vi "7_Hole_Probe Pressures to UVW.vi"() -> ()   [LabVIEW 2017]
uses:
  Controls/Setup.ctl
  Globals/Meas_global.vi
panel:
  out "UVW":dbl[][](array[numeric])
  out "7 Hole Probe chs":string[](array[string])
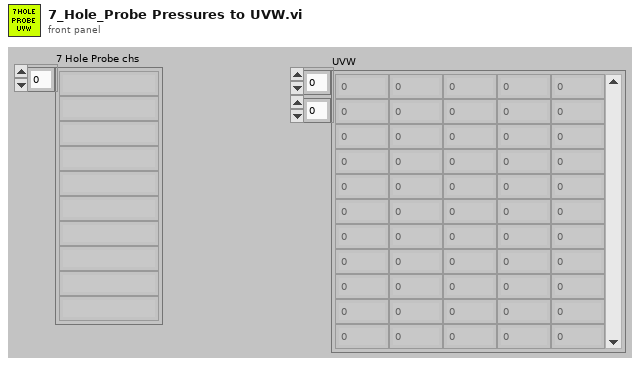
[diagram p1: front panel]
types:
  T1 = typedef "Analysis_info_cluster.ctl" = cluster{"Colour":u32, "Inst type":T2, "Inst name":string, "Symbol":string, "Code name":string, "Extra Info":string, "Inst Array":T3, "Extra Titles":string[], "Extra Values":string[], "U":dbl, "u^2":dbl, "u^3":dbl, "u^4":dbl, "Skew_u":dbl, "Kurt_u":dbl, "Sd Error in Mean":dbl, "% u'/U":dbl, "X":dbl, "Y":dbl, "Z":dbl, "Timescale integral Estimate":dbl, "Sd Error in Variance":dbl, "Calib File":path, "Calib Constants":dbl[], "Output Position":bool, "Full Stats":bool, "Av Sampling Rate":dbl, "Av No of Samples":dbl, "Total Meas Time (s)":dbl, "ADAM Ch Name":string, "Max value":dbl, "Min value":dbl, "Req Sample Rate Hz":dbl, "Sync Delay Time (s)":dbl, "Ch No":i16, "Device ID":string, "Use Latest Calib":bool, "Port":string}
  T2 = typedef "Inst_type.ctl" = enum16{"Propeller anemometer", "Raw voltage", "Pressure Transducer", "Pitot-static tube", "Preston tube", "Hot wire", "Cross wire 1", "Cross wire 2", "Generic Linear", "Generic Polynomial", "Generic BackPoly", "Fast FID", "Thermocouple", "Cold wire", "Pulsed Wire", "LDA Vel", "LDA Tran time", "LDA Arr time", "Microphone"}
  T3 = typedef "Instrument_Array.ctl" = enum16{"PWA", "LDA", "Analogue"}
  T4 = typedef "Time_Trace_Cluster.ctl" = cluster{"Weighting":dbl[], "Time (s)":dbl[], "Voltage":dbl[], "Eng Values":dbl[]}
  T5 = typedef "Setup.ctl" = enum16{"Run Program", "Show Setup", "Save Current Setup", "Setup Front Panel"}
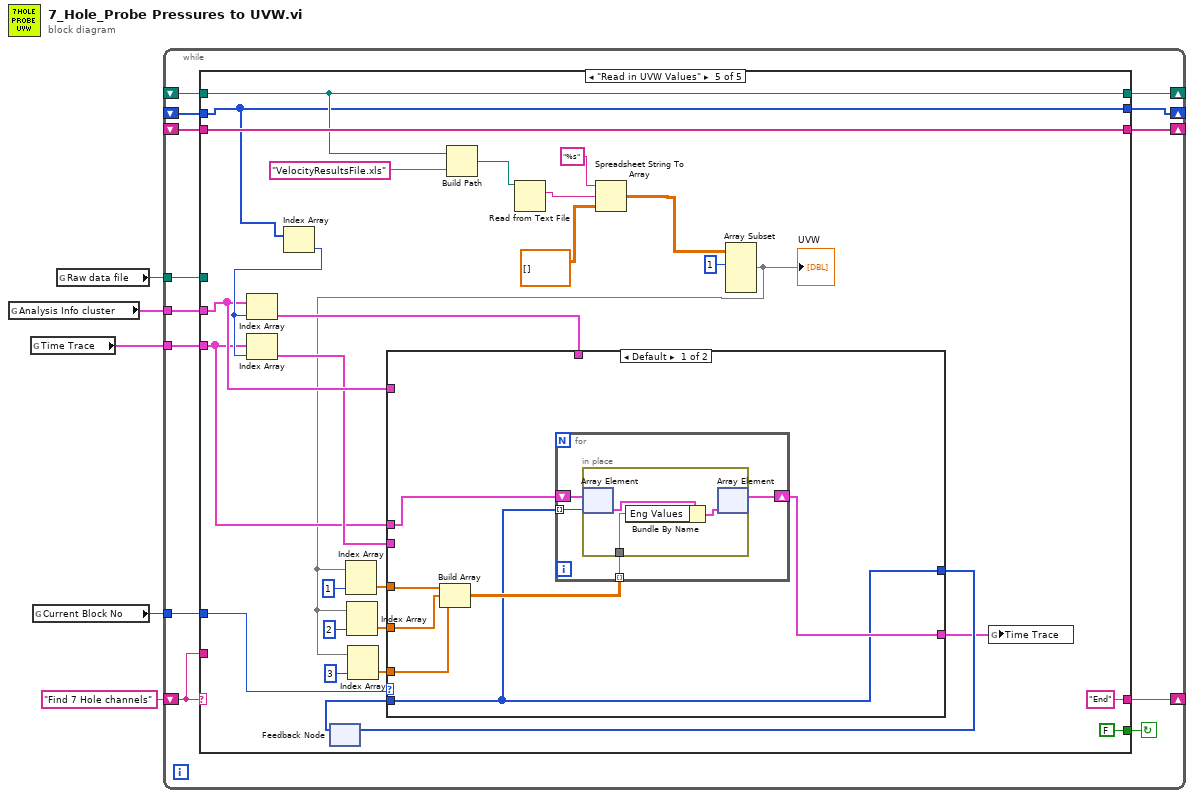
[diagram p0: block diagram]
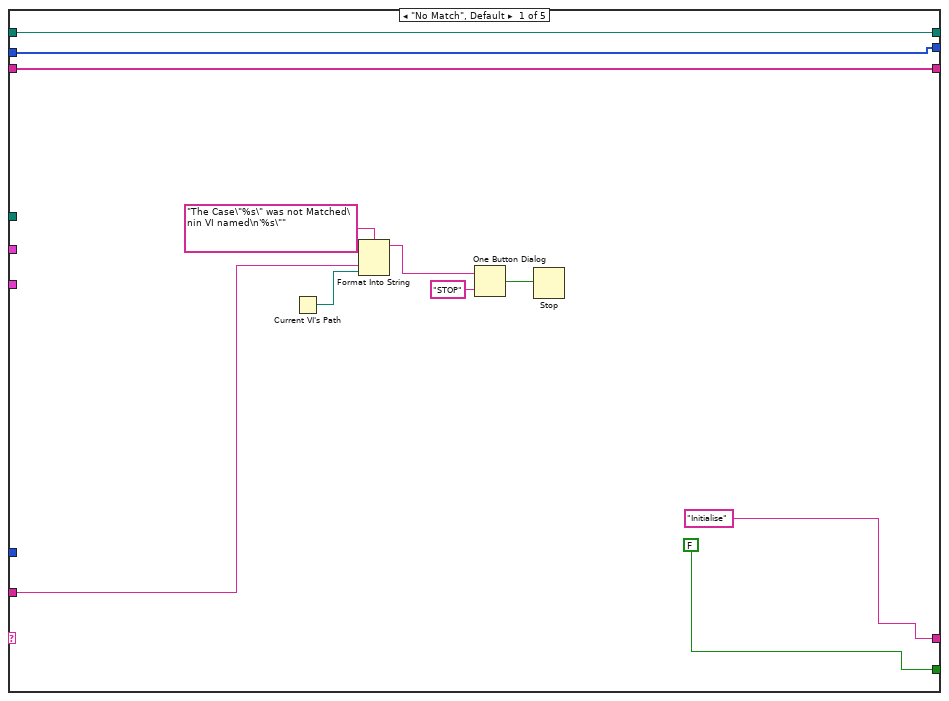
[diagram p2: hidden frame]
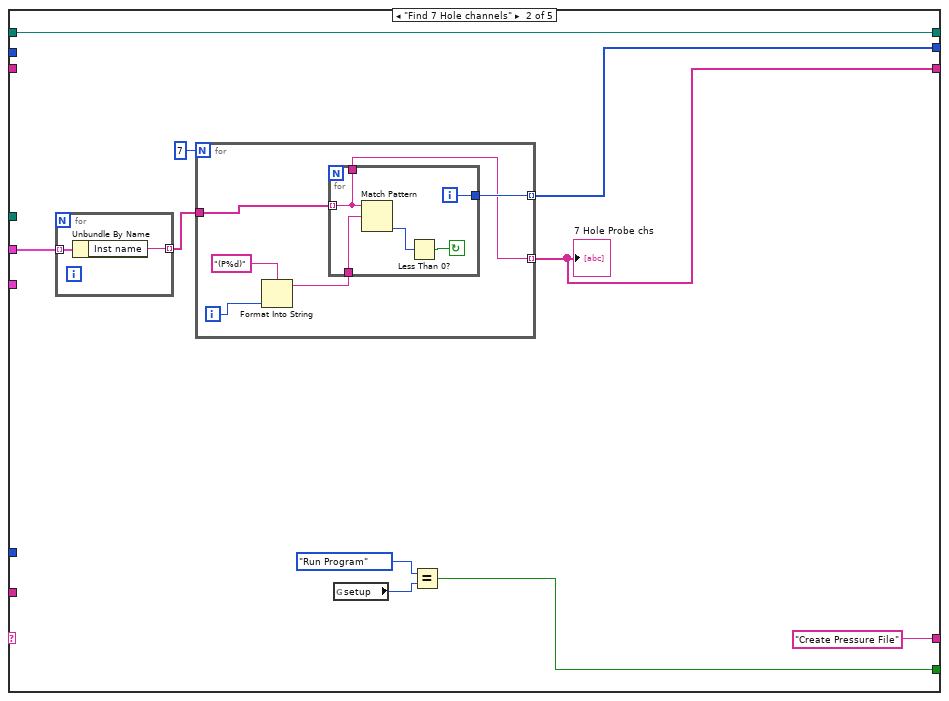
[diagram p3: hidden frame]
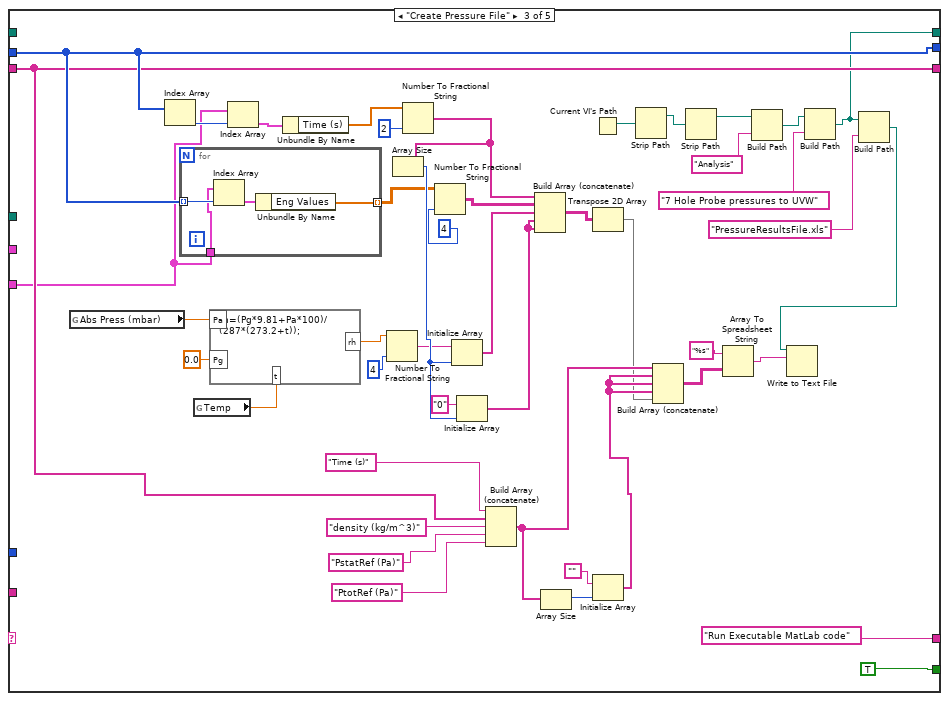
[diagram p4: hidden frame]
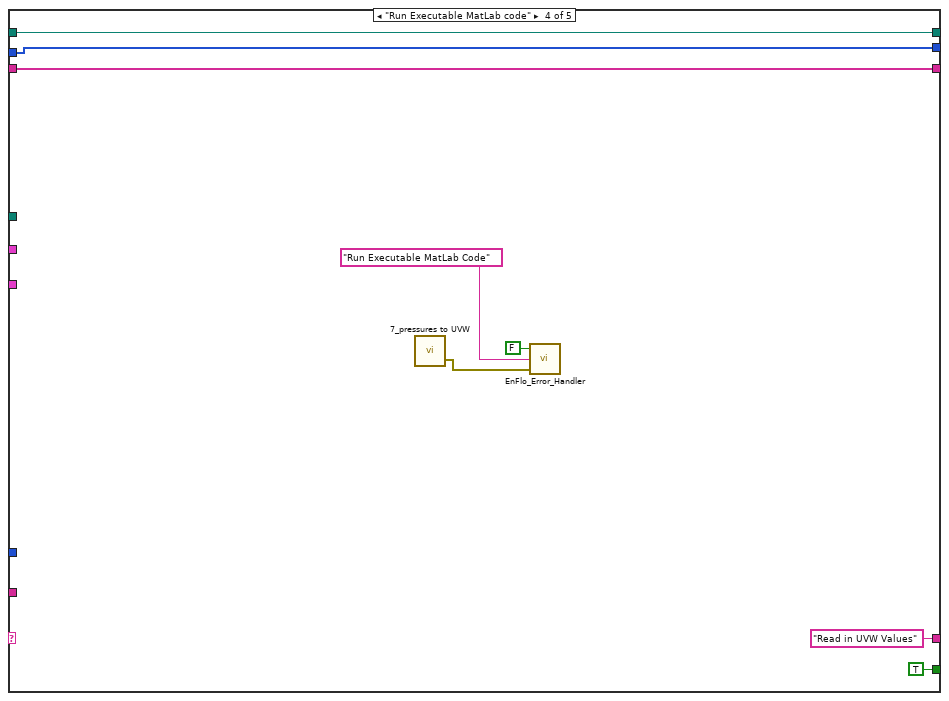
[diagram p5: hidden frame]
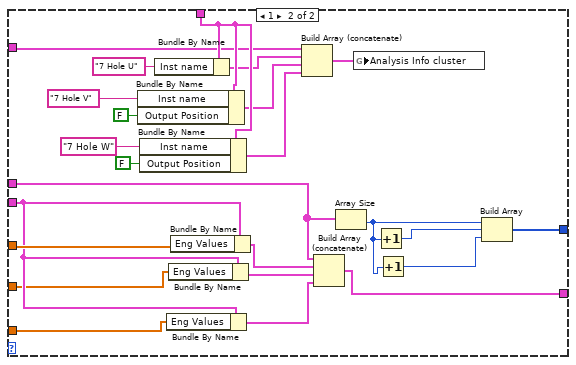
[diagram p6: hidden frame]
diagram:
  n1 = global read "Meas_global.vi" "Analysis Info cluster"() -> (w3:T1[])
  n2 = global read "Meas_global.vi" "Time Trace"() -> (w2:T4[])
  n3 = global read "Meas_global.vi" "Current Block No"() -> (w1:i32)
  n4 = global read "Meas_global.vi" "Raw data file"() -> (w4:path)
  n5 = while {
    shift-left: "Find 7 Hole channels" -> [w16]
    shift-right: [w17] -> _
    tunnel: w4 -> [w15]
    tunnel: w3 -> [w14]
    shift-right: [w13] -> _
    shift-left: _ -> [w12]
    shift-right: [w11] -> _
    shift-left: _ -> [w10]
    shift-right: [w9] -> _
    shift-left: _ -> [w8]
    tunnel: w2 -> [w7]
    tunnel: w1 -> [w6]
    stop <- w18 continue-if-true
    n6 = case shown="\"Read in UVW Values\"" w16 {
      tunnel: [FALSE w30 TRUE TRUE FALSE] -> w18
      tunnel: ["Initialise" "Create Pressure File" ("t") "Run Executable MatLab code" ("t") "Read in UVW Values" ("t") "End" ("t")] -> w17
      tunnel: w16 -> [w24 _ _ _ _]
      tunnel: w15 -> [_ _ _ _ _]
      tunnel: w14 -> [_ w39 _ _ w125]
      tunnel: [w21 w36 w95 w109 w132] -> w13
      tunnel: w12 -> [w21 _ w95 w109 w132]
      tunnel: [w20 w34 w68 w108 w137] -> w11
      tunnel: w10 -> [w20 _ w68 w108 w137]
      tunnel: [w19 w33 w54 w105 w134] -> w9
      tunnel: w8 -> [w19 w33 _ w105 w134]
      tunnel: w7 -> [_ _ w53 _ w115]
      tunnel: w6 -> [_ _ _ _ w114]
      frame "No Match", Default {
        n7 = Current VI's Path() -> (path=w23:path)
        n8 = Format Into String(format string="The Case\"%s\" was not Matched\nin VI named\n'%s\"" ("Format String"), w24, w23) -> (resulting string=w27:string)  [unwired: 2 in, 1 out]
        n9 = One Button Dialog(message=w27, button name ("OK")="STOP") -> (true=w25:bool)
        n10 = Stop(stop? (T)=w25) -> ()
      }
      frame "Find 7 Hole channels" {
        n11 = for {
          tunnel: w39 -> [w52] mode=indexing
          tunnel: [w51] -> w37 mode=indexing
          n12 = Unbundle By Name(w52) -> ("Inst name"=w51:string)
        }
        n13 = for {
          N: 7 -> [_]
          tunnel: w37 -> [w43]
          tunnel: [w41] -> w36 mode=indexing
          tunnel: [w40] -> w34 mode=indexing
          i -> [w45]
          n14 = Format Into String(format string="(P%d)", w45) -> (resulting string=w42:string)  [unwired: 2 in, 1 out]
          n15 = for {
            tunnel: w43 -> [w46] mode=indexing
            tunnel: w42 -> [w50]
            tunnel: [w47] -> w41
            tunnel: [w46] -> w40
            i -> [w47]
            stop <- w49 continue-if-true
            n16 = Match Pattern(string=w46, regular expression=w50) -> (offset past match=w48:i32)  [unwired: 1 in, 3 out]
            n17 = Less Than 0?(x=w48) -> (x < 0?=w49:bool)
          }
        }
        "7 Hole Probe chs" <- w34
        n18 = global read "Meas_global.vi" "setup"() -> (w32:T5)
        n19 = Equal?(x=Setup."Run Program" ("setup"), y=w32) -> (x = y?=w30:bool)
      }
      frame "Create Pressure File" {
        n20 = global read "Meas_global.vi" "Abs Press (mbar)"() -> (w91:dbl)
        n21 = Index Array(array=w95) -> (element=w93:i32)  [unwired: 1 in]
        n22 = for {
          tunnel: w95 -> [w101] mode=indexing
          tunnel: [w98] -> w77 mode=indexing
          tunnel: w53 -> [w99]
          n23 = Index Array(array=w99, index=w101) -> (element=w100:T4)
          n24 = Unbundle By Name(w100) -> ("Eng Values"=w98:dbl[])
        }
        n25 = global read "Meas_global.vi" "Temp"() -> (w92:dbl)
        n26 = formula code="rh=(Pg*9.81+Pa*100)/\n(287*(273.2+t));"("t"=w92, "Pg"=0.0 ("input variable"), "Pa"=w91) -> ("rh"=w74:dbl)
        n27 = Index Array(array=w53, index=w93) -> (element=w94:T4)
        n28 = Unbundle By Name(w94) -> ("Time (s)"=w81:dbl[])
        n29 = Number To Fractional String(number=w74, precision (6)=i16 4) -> (F-format string=w73:string)  [unwired: 2 in]
        n30 = Number To Fractional String(number=w81, precision (6)=i16 2) -> (F-format string=w79:string[])  [unwired: 2 in]
        n31 = Array Size(array=w79) -> (size(s)=w89:i32)
        n32 = Number To Fractional String(number=w77, precision (6)=i16 4) -> (F-format string=w76:string[][])  [unwired: 2 in]
        n33 = Initialize Array(w73, w89) -> (w87:string[])
        n34 = Initialize Array("0" ("element"), w89) -> (w86:string[])
        n35 = Build Array (concatenate)("Time (s)", w68, "density (kg/m^3)", "PstatRef (Pa)", "PtotRef (Pa)") -> (w59:string[])
        n36 = Build Array (concatenate)(w79, w76, w87, w86, w86) -> (w72:string[][])
        n37 = Array Size(array=w59) -> (size(s)=w58:i32)
        n38 = Current VI's Path() -> (path=w67:path)
        n39 = Transpose 2D Array(2D array=w72) -> (transposed array=w55:string[][])
        n40 = Initialize Array("", w58) -> (w56:string[])
        n41 = Strip Path(path=w67) -> (stripped path=w66:path)  [unwired: 1 out]
        n42 = Build Array (concatenate)(w59, w56, w56, w56, w55) -> (w71:string[][])
        n43 = Strip Path(path=w66) -> (stripped path=w65:path)  [unwired: 1 out]
        n44 = Array To Spreadsheet String(array=w71, 3:"%s" ("format string")) -> (spreadsheet string=w69:string)  [unwired: 1 in]
        n45 = Build Path(base path=w65, name or relative path="Analysis") -> (appended path=w63:path)
        n46 = Build Path(base path=w63, name or relative path="7 Hole Probe pressures to UVW") -> (appended path=w54:path)
        n47 = Build Path(base path=w54, name or relative path="PressureResultsFile.xls") -> (appended path=w60:path)
        n48 = Write to Text File(file (use dialog)=w60, text=w69) -> ()  [unwired: 2 in, 3 out]
      }
      frame "Run Executable MatLab code" {
        n49 = call "7_pressures to UVW.vi"() -> ("error out"=w104:errorcluster)  [unwired: 3 in]
        n50 = call "EnFlo_Error_Handler.vi"("error in (no error)"=w104, "Error Type"="Run Executable MatLab Code", "Dialog Box (T)"=FALSE) -> ()  [unwired: 3 out]
      }
      frame "Read in UVW Values" {
        n51 = Index Array(array=w132) -> (element=w127:i32)  [unwired: 1 in]
        n52 = Index Array(array=w125, index=w127) -> (element=w126:T1)
        n53 = Index Array(array=w115, index=w127) -> (element=w124:T4)
        n54 = feedback #1() -> (w111:i32[])  [unwired: 1 in]
        n55 = Build Path(base path=w134, name or relative path="VelocityResultsFile.xls") -> (appended path=w131:path)
        n56 = Read from Text File(file (use dialog)=w131) -> (text=w130:string)  [unwired: 3 in, 3 out]
        n57 = Spreadsheet String To Array(format string="%s", spreadsheet string=w130, array type (2D Dbl)=dbl[][] []) -> (array=w123:dbl[][])  [unwired: 1 in]
        n58 = Array Subset(array=w123, index (row)=1 ("index")) -> (w113:dbl[][])  [unwired: 3 in]
        "UVW" <- w113
        n59 = Index Array(array=w113, index (col)=1 ("disabled index (col)")) -> (element=w118:dbl[])  [unwired: 1 in]
        n60 = Index Array(array=w113, index (col)=2 ("disabled index (col)")) -> (element=w117:dbl[])  [unwired: 1 in]
        n61 = Index Array(array=w113, index (col)=3 ("disabled index (col)")) -> (element=w116:dbl[])  [unwired: 1 in]
        n62 = case shown="Default" w114 {
          tunnel: w126 -> [_ w172]
          tunnel: w125 -> [_ w171]
          tunnel: w124 -> [_ w165]
          tunnel: w118 -> [w142 w166]
          tunnel: w117 -> [w141 w164]
          tunnel: w116 -> [w140 w163]
          tunnel: w115 -> [w144 w157]
          tunnel: [w138 w153] -> w112
          tunnel: w111 -> [w138 _]
          tunnel: [w143 w152] -> w110
          frame Default {
            n63 = Build Array(w142, w141, w140) -> (w139:dbl[][])
            n64 = for {
              tunnel: w138 -> [w148] mode=indexing
              shift-right: [w146] -> w143
              shift-left: w144 -> [w147]
              tunnel: w139 -> [w145] mode=indexing
              n65 = in-place {
                in-place-border: w145 -> [w149]
                n66 = in-place-array #2(w147, w148) -> (w151:T4)
                n67 = Bundle By Name(cluster=w151, "Eng Values"=w149) -> (w150:T4)
                n68 = in-place-array #2(w150) -> (w146:T4[])  [unwired: 1 out]
              }
            }
          }
          frame 1 {
            n69 = Bundle By Name(cluster=w172, "Inst name"="7 Hole V", "Output Position"=FALSE) -> (w169:T1)
            n70 = Bundle By Name(cluster=w172, "Inst name"="7 Hole W", "Output Position"=FALSE) -> (w168:T1)
            n71 = Bundle By Name(cluster=w172, "Inst name"="7 Hole U") -> (w170:T1)
            n72 = Bundle By Name(cluster=w165, "Eng Values"=w163) -> (w160:T4)
            n73 = Bundle By Name(cluster=w165, "Eng Values"=w164) -> (w161:T4)
            n74 = Bundle By Name(cluster=w165, "Eng Values"=w166) -> (w162:T4)
            n75 = Build Array (concatenate)(w171, w170, w169, w168) -> (w167:T1[])
            n76 = Build Array (concatenate)(w157, w162, w161, w160) -> (w152:T4[])
            n77 = Array Size(array=w157) -> (size(s)=w155:i32)
            n78 = global write "Meas_global.vi" "Analysis Info cluster"(w167) -> ()
            n79 = Increment(x=w155) -> (x+1=w156:i32)
            n80 = Increment(x=w155) -> (x+1=w154:i32)
            n81 = Build Array(w155, w156, w154) -> (w153:i32[])
          }
        }
        n82 = feedback-in #1(w112) -> ()
        n83 = global write "Meas_global.vi" "Time Trace"(w110) -> ()
      }
    }
  }
